vi "Configure Output Limits.vi"(0 "VISA resource name":refnum<visa-resource-name>, 1 "Unit Address (1)":u8=1 min=1 max=254, 7 "Type of Limit (0:Low)":u16(ring) items=["Low", "High"], 9 "Output Limit Value (0)":sgl min=-100 max=100 format="%.2g", 11 "error in (no error)":errorcluster) -> (4 "VISA resource name out":refnum<visa-resource-name>, 15 "error out":errorcluster)   [LabVIEW 2010, in "Eurotherm 32xx Series.lvlib"]
doc: "This VI sets Output limits.\n\nDescription:\n\nMaximum-\nMaximum output power delivered by channels 1 and 2.\nBy reducing the high power limit, it is possible to reduce the rate of change of the process, however, care should be taken as reducing the power limit will reduce the controllers ability to react to disturbance.\n\nMinimum-\nMinimum (or maximum negative) output power delivered by channels 1 and 2.\nFor a 1 channel (heat only) algorithm this value will typically be set to 0%\nFor a 2 channel (heat/cool) algorithm this value will typically be set to -100%"
uses:
  <instrlib>/Eurotherm 32xx Series/Eurotherm 32xx Series.lvlib
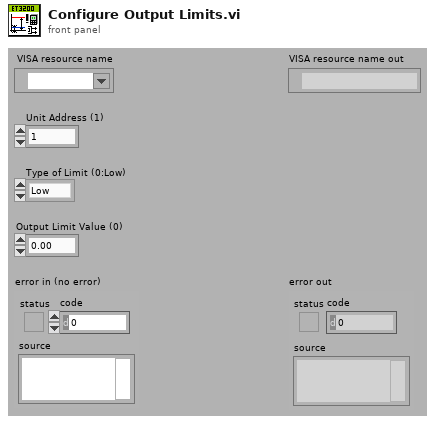
[diagram p1: front panel]
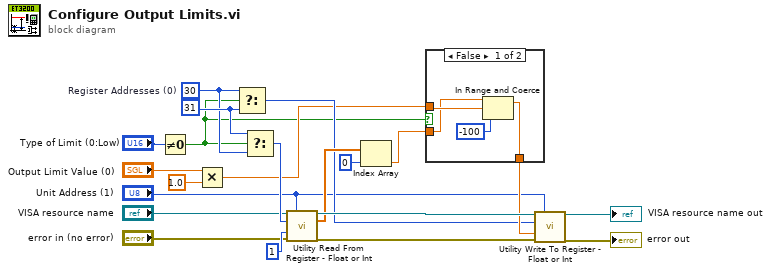
[diagram p0: block diagram]
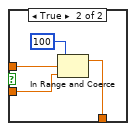
[diagram p2: hidden frame]
diagram:
  w18 = u16 31 ("Register Addresses (0)")
  w17 = u16 30  # Register Addresses (0)
  n1 = Not Equal To 0?(x="Type of Limit (0:Low)") -> (x != 0?=w1:bool)
  n2 = Multiply(x="Output Limit Value (0)", y=sgl 1.0) -> (x*y=w4:sgl)
  n3 = Select(t=w17, s=w1, f=w18) -> (s? t:f=w11:u16)
  n4 = Select(t=w18, s=w1, f=w17) -> (s? t:f=w16:u16)
  n5 = call <instrlib>:"Utility Read From Register - Float or Int.vi"("VISA resource name"="VISA resource name", "Unit Address (1)"="Unit Address (1)", "Register Address (0)"=w16, "Num Of Reg (1)"=u16 1, "error in (no error)"="error in (no error)") -> ("VISA resource name out"=w21:refnum<visa-resource-name>, "Data"=w15:sgl[], "error out"=w20:errorcluster)  [unwired: 8 in]
  n6 = Index Array(array=w15, index=0) -> (element=w13:sgl)
  n7 = case shown="False" w1 {
    tunnel: w13 -> [w23 w28]
    tunnel: w4 -> [w25 w27]
    tunnel: [w22 w26] -> w12
    frame False {
      n8 = In Range and Coerce(upper limit=w23, x=w25, lower limit=-100 ("upper limit")) -> (coerced(x)=w22:sgl)  [unwired: 1 out]
    }
    frame True {
      n9 = In Range and Coerce(upper limit=100, x=w27, lower limit=w28) -> (coerced(x)=w26:sgl)  [unwired: 1 out]
    }
  }
  n10 = call <instrlib>:"Utility Write To Register - Float or Int.vi"("VISA resource name"=w21, "Unit Address (1)"="Unit Address (1)", "Register Address (0)"=w11, "Data (0)"=w12, "error in (no error)"=w20) -> ("VISA resource name out"=→"VISA resource name out":refnum<visa-resource-name>, "error out"=→"error out":errorcluster)  [unwired: 9 in]
